vi "motor_control.vi"() -> ()   [LabVIEW 2009]
uses:
  <vilib>/Platform/TimedLoop/XDataNode/wakeup.ctl
  <vilib>/Platform/TimedLoop/XDataNode/XDNodeRunTimeDep.lvlib
  <vilib>/Platform/TimedLoop/XDataNode/nitl_modes.ctl
  <vilib>/Platform/TimedLoop/XDataNode/timing_clust.ctl
  <vilib>/Platform/TimedLoop/XDataNode/XDataNode.xnode
  <vilib>/eio/EIONode/EIONode.xnode
  <vilib>/Platform/TimedLoop/XDataNode/loadlvalarms.vi
  <vilib>/rvi/eio/nirviEIOImplementation/nirviEIOImplementation.xnode
  <vilib>/rvi/eio/common/nirviEmuTemplateMethod_noerrors.vi
  <vilib>/rvi/eio/common/nirviEmuClasses.ctl
  <vilib>/addons/control/pid/fpga.llb/XNode/niFpgaPID.xnode
panel:
  out "Wheel Position":i32
  in  "M1 Reset Position":bool
  in  "M1 Reset Position Value":i32
  out "M1 Encoder Position":i32
  out "M1 ticks/count":u32
  out "M1 Index (Z) Position":i32
  out "M1 counts (no reset)":i32
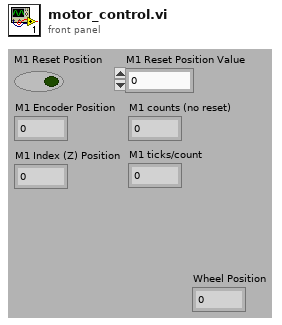
[diagram p1: front panel]
types:
  T1 = typedef "XDNodeRunTimeDep.lvlib/timing_clust.ctl" = cluster{"Expected End [f-1]":u64, "Actual End [f-1]":u64, "Finished Late? [f-1]":bool, "Expected End [i-1]":u64, "Actual End [i-1]":u64, "Finished Late? [i-1]":bool, "Expected Start [i]":u64, "Actual Start [i]":u64, "Expected Start [f]":u64, "Actual Start [f]":u64, "Source Name":string, "Structure Name":string, "Period":i64, "Deadline":i64, "Offset":i64, "Start":i64, "Priority":i32, "Timeout":i32, "Mode":T2, "Wakeup Reason":T3, "Error":errorcluster, "Source Type":string, "Secondary Source Type":string, "Global End Time":u64, "Global Start Time":u64, "Frame Duration":u64, "Iteration Duration":u64, "Assigned CPU":i32, "I/O Scan Engine Mode":u32}
  T2 = typedef "XDNodeRunTimeDep.lvlib/nitl_modes.ctl" = enum32{"No Change", "Process missed periods, maintain original phase", "Discard missed periods, maintain original phase", "Process missed periods, ignore original phase", "Discard missed periods, ignore original phase"}
  T3 = typedef "XDNodeRunTimeDep.lvlib/wakeup.ctl" = enum32{"Normal", "Aborted", "Asynchronous wakeup", "Timing source error", "Timed loop error", "Timeout"}
  T4 = typedef "nirviEmuClasses.ctl" = enum16{"IO Read", "IO Write", "Method", "Property Read", "Property Write"}
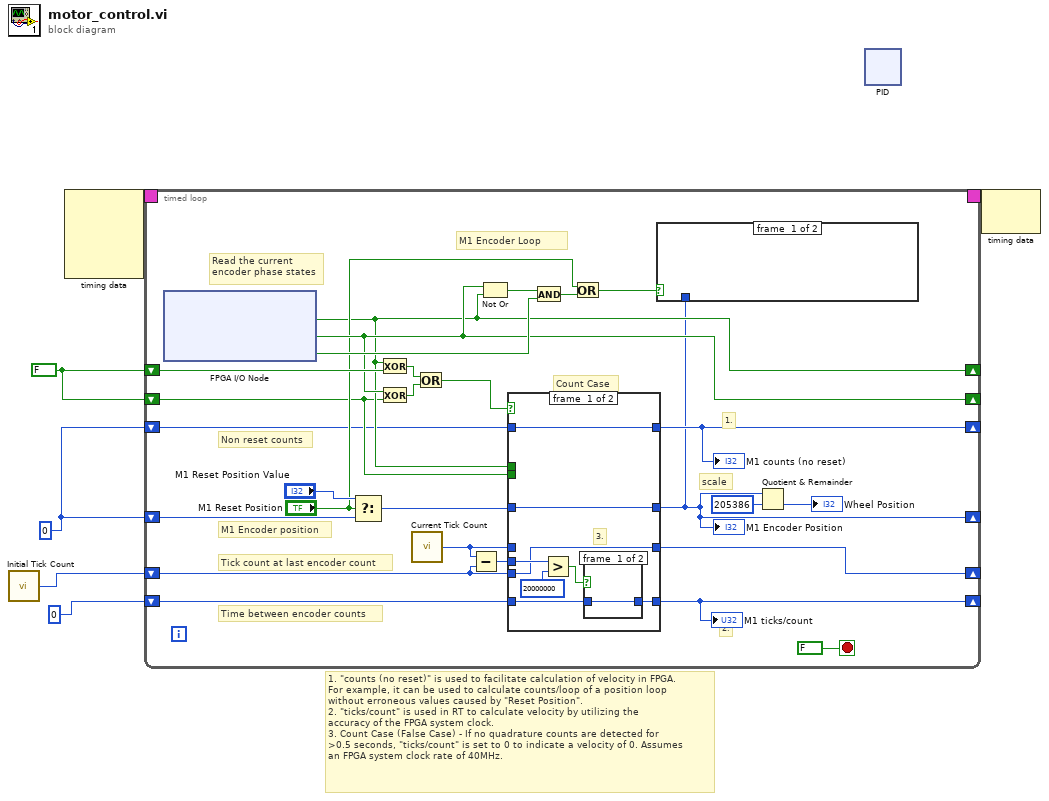
[diagram p0: block diagram]
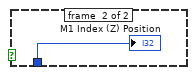
[diagram p2: hidden frame]
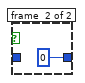
[diagram p3: hidden frame]
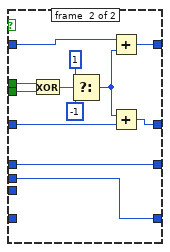
[diagram p4: hidden frame]
diagram:
  w1 = 0 ("Reset Position Value")
  w4 = FALSE ("Encoder Phase A")
  # "1. \"counts (no reset)\" is used to facilitate calculation of velocity in FPGA.\nFor example, it can be used to calculate counts/loop of a position loop\nwithout erroneous values caused by \"Reset Position\". \n2. \"ticks/count\" is used in RT to calculate velocity by utilizing the\naccuracy of the FPGA system clock.\n3. Count Case (False Case) - If no quadrature counts are detected for\n>0.5 seconds, \"ticks/count\" is set to 0 to indicate a velocity of 0. Assumes\nan FPGA system clock rate of 40MHz."
  n1 = call "Initial Tick Count"() -> ("Tick Count(Ticks)"=w3:u32)
  n2 = node-c288() -> (w6:T1)  [unwired: 4 in]
  n3 = timed-loop {
    shift-right: [w16] -> _
    shift-left: w4 -> [w33]
    shift-right: [w21] -> _
    shift-left: w4 -> [w15]
    shift-right: [w8] -> _
    shift-left: w1 -> [w30]
    shift-right: [w26] -> _
    shift-left: w3 -> [w11]
    shift-right: [w25] -> _
    shift-left: u32 0 -> [w24]
    timing: w6 -> [_]
    timing-out: [_] -> w5
    shift-right: [w13] -> _
    shift-left: w1 -> [w14]
    stop <- FALSE stop-if-true
    # "scale"
    # "Count Case"
    # "M1 Encoder Loop"
    # "2."
    # "1."
    # "Read the current\nencoder phase states"
    # "Non reset counts"
    # "M1 Encoder position"
    # "Time between encoder counts"
    # "Tick count at last encoder count"
    n4 = xnode "FPGA I/O Node"() -> ("M1_encoder_PhaseA"=w16:bool, "M1_encoder_PhaseB"=w21:bool, "M1_encoder_index"=w22:bool)  [unwired: 3 in, 3 out]
    n5 = Select(t="M1 Reset Position Value", s="M1 Reset Position", f=w30) -> (s? t:f=w28:i32)
    n6 = Exclusive Or(1:w33, 2:w16) -> (0:w32:bool)
    n7 = Exclusive Or(1:w15, 2:w21) -> (0:w31:bool)
    n8 = call "Current Tick Count"() -> ("Tick Count(Ticks)"=w12:u32)
    n9 = Or(x=w32, y=w31) -> (x .or. y?=w29:bool)
    n10 = Subtract(x=w12, y=w11) -> (x-y=w10:u32)
    n11 = Not Or(1:w16, 2:w21) -> (0:w19:bool)
    n12 = case shown="False" w29 {
      tunnel: [w42 w50] -> w8
      tunnel: w28 -> [w42 w56]
      tunnel: w12 -> [_ w46]
      tunnel: [w37 w46] -> w26
      tunnel: w11 -> [w37 _]
      tunnel: [w35 w45] -> w25
      tunnel: w24 -> [w36 _]
      tunnel: w16 -> [_ w52]
      tunnel: w15 -> [_ w51]
      tunnel: [w41 w48] -> w13
      tunnel: w14 -> [w41 w47]
      tunnel: w10 -> [w38 w45]
      frame #0 {
        # "3."
        n13 = Greater?(x=w38, y=u32 20000000 ("x")) -> (0:w39:bool)
        n14 = case shown="False" w39 {
          tunnel: [w43 u32 0] -> w35
          tunnel: w36 -> [w43 _]
          frame #0 {
          }
          frame #1 {
          }
        }
      }
      frame #1 {
        n15 = Exclusive Or(1:w51, 2:w52) -> (0:w53:bool)
        n16 = Select(t=1 ("16 bit"), s=w53, f=-1 ("16 bit")) -> (s? t:f=w49:i32)
        n17 = Add(x=w47, y=w49) -> (x+y=w48:i32)
        n18 = Add(x=w49, y=w56) -> (x+y=w50:i32)
      }
    }
    "M1 Encoder Position" <- w8
    "M1 ticks/count" <- w25
    "M1 counts (no reset)" <- w13
    n19 = And(x=w19, y=w22) -> (x .and. y?=w20:bool)
    n20 = Or(x="M1 Reset Position", y=w20) -> (x .or. y?=w18:bool)
    n21 = case shown="True" w18 {
      tunnel: w8 -> [_ w34]
      frame #0 {
      }
      frame #1 {
        "M1 Index (Z) Position" <- w34
      }
    }
    n22 = Quotient & Remainder(x=w8, y=205386) -> (floor(x/y)=→"Wheel Position":i32)  [unwired: 1 out]
  }
  n23 = xnode ("PID")() -> ()  [unwired: 5 in, 1 out]
  n24 = node-c288(w5) -> ()  [unwired: 1 out]
